vi "Camera Begin.vi"() -> ()   [LabVIEW 2013]
uses:
  <vilib>/Rock Robotics/WPI/Camera/WPI_CameraWhite Balance Values.ctl
  <vilib>/Rock Robotics/WPI/Camera/WPI_CameraFrameRate.ctl
  <vilib>/Rock Robotics/WPI/Camera/WPI_CameraExposure Values.ctl
  <vilib>/Rock Robotics/WPI/Camera/WPI_CameraImageSize.ctl
panel:
  in  "Camera 2":T5={"Camera Address"="192.168.0.90", "Compression"=0, "White Balance"=enum."Auto", "Frame Rate (fps)"=30, "Exposure"=enum."Auto", "Image Size"=enum."320x240", "Brightness"=50, "refnum name"="My Camera RefNum"} {"Brightness" min=0 max=100; "Frame Rate (fps)" min=1 max=30; "Compression" min=0 max=100}
  in  "Camera 1":T5={"Camera Address"="192.168.0.90", "Compression"=0, "White Balance"=enum."Auto", "Frame Rate (fps)"=30, "Exposure"=enum."Auto", "Image Size"=enum."320x240", "Brightness"=50, "refnum name"="My Camera RefNum"} {"Brightness" min=0 max=100; "Frame Rate (fps)" min=1 max=30; "Compression" min=0 max=100}
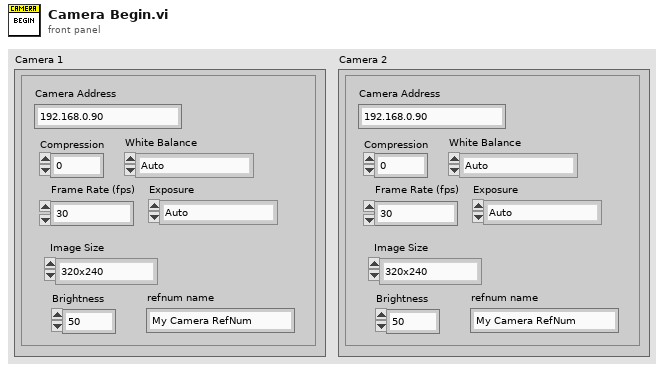
[diagram p1: front panel]
types:
  T1 = typedef "WPI_CameraWhite Balance Values.ctl" = enum16{"Auto", "Fixed indoor", "Fixed outdoor 1", "Fixed outdoor 2", "Fixed fluorescent 1", "Fixed fluorescent 2", "Hold current"}
  T2 = typedef "WPI_CameraFrameRate.ctl" = u32
  T3 = typedef "WPI_CameraExposure Values.ctl" = enum16{"Auto", "Flicker-free 50 Hz", "Flicker-free 60 Hz", "Hold current"}
  T4 = typedef "WPI_CameraImageSize.ctl" = enum16{"640x480", "320x240", "160x120"}
  T5 = cluster{"Camera Address":string, "Compression":i32, "White Balance":T1, "Frame Rate (fps)":T2, "Exposure":T3, "Image Size":T4, "Brightness":i32, "refnum name":string}
  T6 = typedef "WPI_CameraDevRef.ctl" = cluster{"Camera Address":string, "CameraStatus":errorcluster, "Acquire Image Notifier":refnum<notifier>}
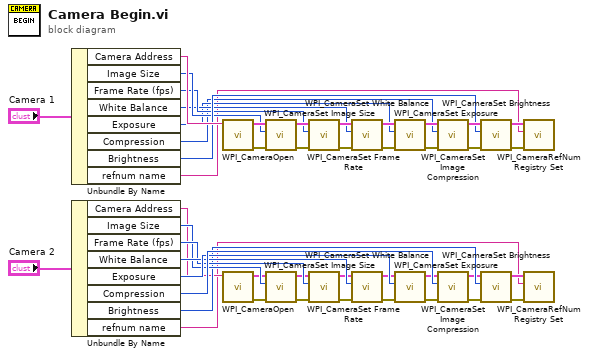
[diagram p0: block diagram]
diagram:
  n1 = Unbundle By Name("Camera 1") -> ("Camera Address"=w31:string, "Image Size"=w29:T4, "Frame Rate (fps)"=w28:T2, "White Balance"=w27:T1, "Exposure"=w26:T3, "Compression"=w25:i32, "Brightness"=w30:i32, "refnum name"=w2:string)
  n2 = Unbundle By Name("Camera 2") -> ("Camera Address"=w18:string, "Image Size"=w20:T4, "Frame Rate (fps)"=w21:T2, "White Balance"=w22:T1, "Exposure"=w23:T3, "Compression"=w24:i32, "Brightness"=w19:i32, "refnum name"=w1:string)
  n3 = call <vilib>:"WPI_CameraOpen.vi"("Camera Address"=w31) -> ("error out"=w40:errorcluster, "CameraDevRef"=w41:T6)  [unwired: 1 in, 8 out]
  n4 = call <vilib>:"WPI_CameraOpen.vi"("Camera Address"=w18) -> ("error out"=w9:errorcluster, "CameraDevRef"=w8:T6)  [unwired: 1 in, 8 out]
  n5 = call <vilib>:"WPI_CameraSet Image Size.vi"("error in (no error)"=w40, "Image Size"=w29, "CameraDevRef"=w41) -> ("error out"=w39:errorcluster, "CameraDevRef Out"=w42:T6)  [unwired: 7 out]
  n6 = call <vilib>:"WPI_CameraSet Image Size.vi"("error in (no error)"=w9, "Image Size"=w20, "CameraDevRef"=w8) -> ("error out"=w10:errorcluster, "CameraDevRef Out"=w7:T6)  [unwired: 7 out]
  n7 = call <vilib>:"WPI_CameraSet Frame Rate.vi"("error in (no error)"=w39, "Frame Rate (fps)"=w28, "CameraDevRef"=w42) -> ("error out"=w38:errorcluster, "CameraDevRef Out"=w44:T6)  [unwired: 7 out]
  n8 = call <vilib>:"WPI_CameraSet Frame Rate.vi"("error in (no error)"=w10, "Frame Rate (fps)"=w21, "CameraDevRef"=w7) -> ("error out"=w11:errorcluster, "CameraDevRef Out"=w5:T6)  [unwired: 7 out]
  n9 = call <vilib>:"WPI_CameraSet White Balance.vi"("error in (no error)"=w38, "White Balance"=w27, "CameraDevRef"=w44) -> ("error out"=w37:errorcluster, "CameraDevRef Out"=w43:T6)  [unwired: 7 out]
  n10 = call <vilib>:"WPI_CameraSet White Balance.vi"("error in (no error)"=w11, "White Balance"=w22, "CameraDevRef"=w5) -> ("error out"=w12:errorcluster, "CameraDevRef Out"=w6:T6)  [unwired: 7 out]
  n11 = call <vilib>:"WPI_CameraSet Exposure.vi"("error in (no error)"=w37, "Exposure"=w26, "CameraDevRef"=w43) -> ("error out"=w36:errorcluster, "CameraDevRef Out"=w46:T6)  [unwired: 7 out]
  n12 = call <vilib>:"WPI_CameraSet Exposure.vi"("error in (no error)"=w12, "Exposure"=w23, "CameraDevRef"=w6) -> ("error out"=w13:errorcluster, "CameraDevRef Out"=w3:T6)  [unwired: 7 out]
  n13 = call <vilib>:"WPI_CameraSet Image Compression.vi"("error in (no error)"=w36, "Compression"=w25, "CameraDevRef"=w46) -> ("error out"=w35:errorcluster, "CameraDevRef Out"=w45:T6)  [unwired: 7 out]
  n14 = call <vilib>:"WPI_CameraSet Image Compression.vi"("error in (no error)"=w13, "Compression"=w24, "CameraDevRef"=w3) -> ("error out"=w14:errorcluster, "CameraDevRef Out"=w4:T6)  [unwired: 7 out]
  n15 = call <vilib>:"WPI_CameraSet Brightness.vi"("error in (no error)"=w35, "Brightness"=w30, "CameraDevRef"=w45) -> ("error out"=w33:errorcluster, "CameraDevRef Out"=w34:T6)  [unwired: 7 out]
  n16 = call <vilib>:"WPI_CameraSet Brightness.vi"("error in (no error)"=w14, "Brightness"=w19, "CameraDevRef"=w4) -> ("error out"=w16:errorcluster, "CameraDevRef Out"=w15:T6)  [unwired: 7 out]
  n17 = call <vilib>:"WPI_CameraRefNum Registry Set.vi"("error in (no error)"=w33, "refnum name"=w2, "CameraDevRef"=w34) -> ()  [unwired: 9 out]
  n18 = call <vilib>:"WPI_CameraRefNum Registry Set.vi"("error in (no error)"=w16, "refnum name"=w1, "CameraDevRef"=w15) -> ()  [unwired: 9 out]
